vi "swerveeficncy.vi"() -> ()   [LabVIEW 2017]
panel:
  out "reverse":bool=TRUE
  out "setpoint":dbl
  in  "sp":dbl
  in  "pv":dbl
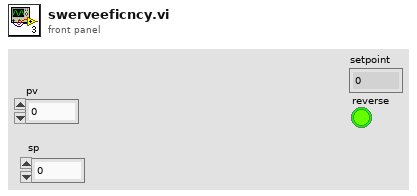
[diagram p1: front panel]
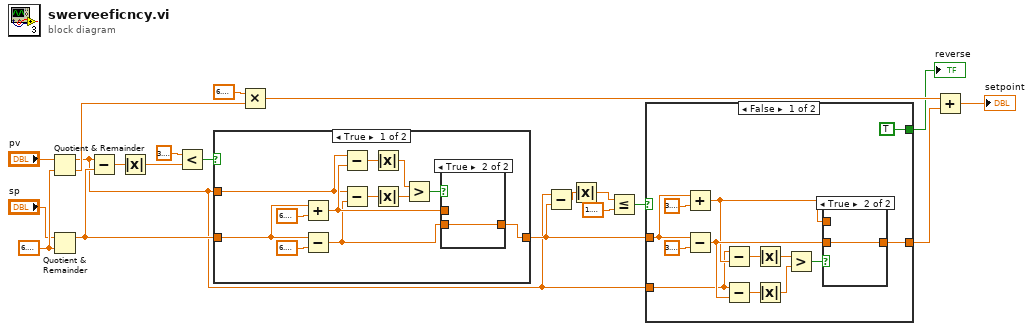
[diagram p0: block diagram]
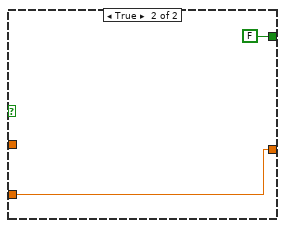
[diagram p3: hidden frame]
diagram:
  w19 = 6.283185307179586
  n1 = Quotient & Remainder(x="pv", y=w19) -> (x-y*floor(x/y)=w3:dbl, floor(x/y)=w17:dbl)
  n2 = Quotient & Remainder(x="sp", y=w19) -> (x-y*floor(x/y)=w13:dbl)  [unwired: 1 out]
  n3 = Subtract(x=w3, y=w13) -> (x-y=w14:dbl)
  n4 = Absolute Value(x=w14) -> (abs(x)=w10:dbl)
  n5 = Less?(x=3.141592653589793, y=w10) -> (x < y?=w12:bool)
  n6 = case shown="True" w12 {
    tunnel: w13 -> [w23 w35]
    tunnel: w3 -> [w22 _]
    tunnel: [w21 w35] -> w4
    frame True {
      n7 = Add(x=w23, y=6.283185307179586) -> (x+y=w32:dbl)
      n8 = Subtract(x=w23, y=6.283185307179586) -> (x-y=w31:dbl)
      n9 = Subtract(x=w22, y=w32) -> (x-y=w26:dbl)
      n10 = Subtract(x=w22, y=w31) -> (x-y=w27:dbl)
      n11 = Absolute Value(x=w26) -> (abs(x)=w28:dbl)
      n12 = Absolute Value(x=w27) -> (abs(x)=w29:dbl)
      n13 = Greater?(x=w28, y=w29) -> (0:w30:bool)
      n14 = case shown="True" w30 {
        tunnel: [w33 w34] -> w21
        tunnel: w31 -> [_ w34]
        tunnel: w32 -> [w33 _]
        frame False {
        }
        frame True {
        }
      }
    }
    frame False {
    }
  }
  n15 = Multiply(x=6.283185307179586, y=w17) -> (x*y=w16:dbl)
  n16 = Subtract(x=w3, y=w4) -> (x-y=w2:dbl)
  n17 = Absolute Value(x=w2) -> (abs(x)=w1:dbl)
  n18 = Less Or Equal?(x=w1, y=1.5707963267948966) -> (x <= y?=w7:bool)
  n19 = case shown="False" w7 {
    tunnel: w3 -> [w39 w51]
    tunnel: w4 -> [w38 _]
    tunnel: [TRUE FALSE] -> w6
    tunnel: [w36 w51] -> w5
    frame False {
      n20 = Add(x=w38, y=3.141592653589793) -> (x+y=w40:dbl)
      n21 = Subtract(x=w38, y=3.141592653589793) -> (x-y=w41:dbl)
      n22 = Subtract(x=w39, y=w40) -> (x-y=w46:dbl)
      n23 = Subtract(x=w39, y=w41) -> (x-y=w45:dbl)
      n24 = Absolute Value(x=w46) -> (abs(x)=w44:dbl)
      n25 = Absolute Value(x=w45) -> (abs(x)=w43:dbl)
      n26 = Greater?(x=w44, y=w43) -> (0:w42:bool)
      n27 = case shown="True" w42 {
        tunnel: [w49 w50] -> w36
        tunnel: w41 -> [_ w50]
        tunnel: w40 -> [w49 _]
        frame False {
        }
        frame True {
        }
      }
    }
    frame True {
    }
  }
  "reverse" <- w6
  n28 = Add(x=w16, y=w5) -> (x+y=→"setpoint":dbl)
